vi "DAQmx_CreateAnalogPuls.vi"(0 "physical channel":string[](array[string])=["Dev1/ao0"], 5 "data":dbl[][](array[numeric]) format="%0.2f", 7 "rate":dbl=1000000.0, 11 "error in":errorcluster) -> (4 "task out":refnum<k21>, 15 "error out":errorcluster)   [LabVIEW 2010]
uses:
  <vilib>/DAQmx/write.llb/DAQmx Write.vi
  <vilib>/DAQmx/write.llb/DAQmx Write (Analog 2D DBL NChan NSamp).vi
  <vilib>/DAQmx/configure/timing.llb/DAQmx Timing (Sample Clock).vi
  <vilib>/DAQmx/configure/trigger.llb/DAQmx Trigger.vi
  <vilib>/DAQmx/configure/trigger.llb/DAQmx Start Trigger (Digital Edge).vi
  <vilib>/DAQmx/create/channels.llb/DAQmx Create Channel (AO-Voltage-Basic).vi
  <vilib>/daqmx/miscellaneous.llb/DAQmx Fill In Error Info.vi
  Program Files/National Instruments/LabVIEW 2010/resource/objmgr/daqmx.rc
panel:
  in  "timeout (s)":dbl=10.0 format="%0.2f"
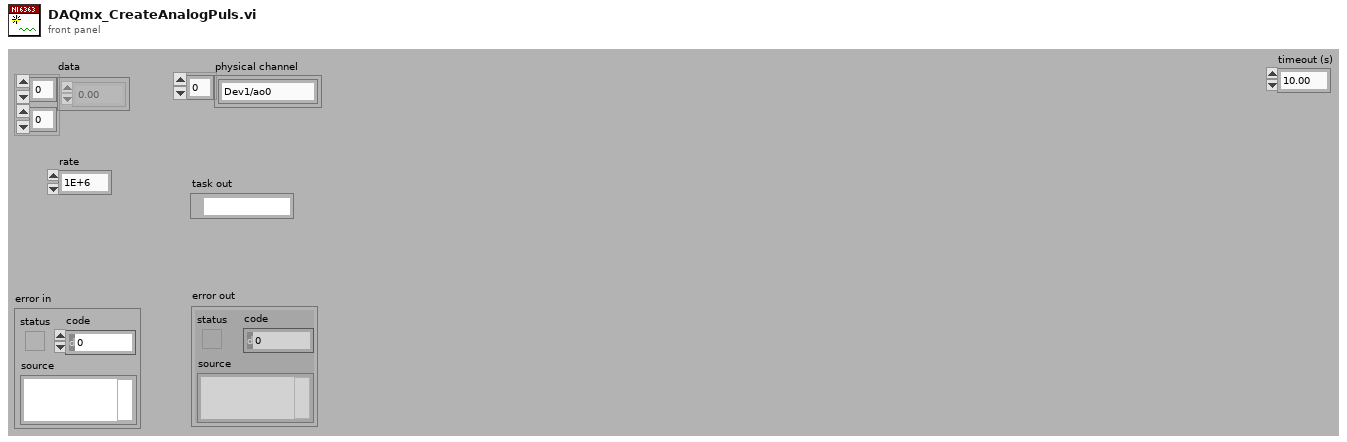
[diagram p1: front panel]
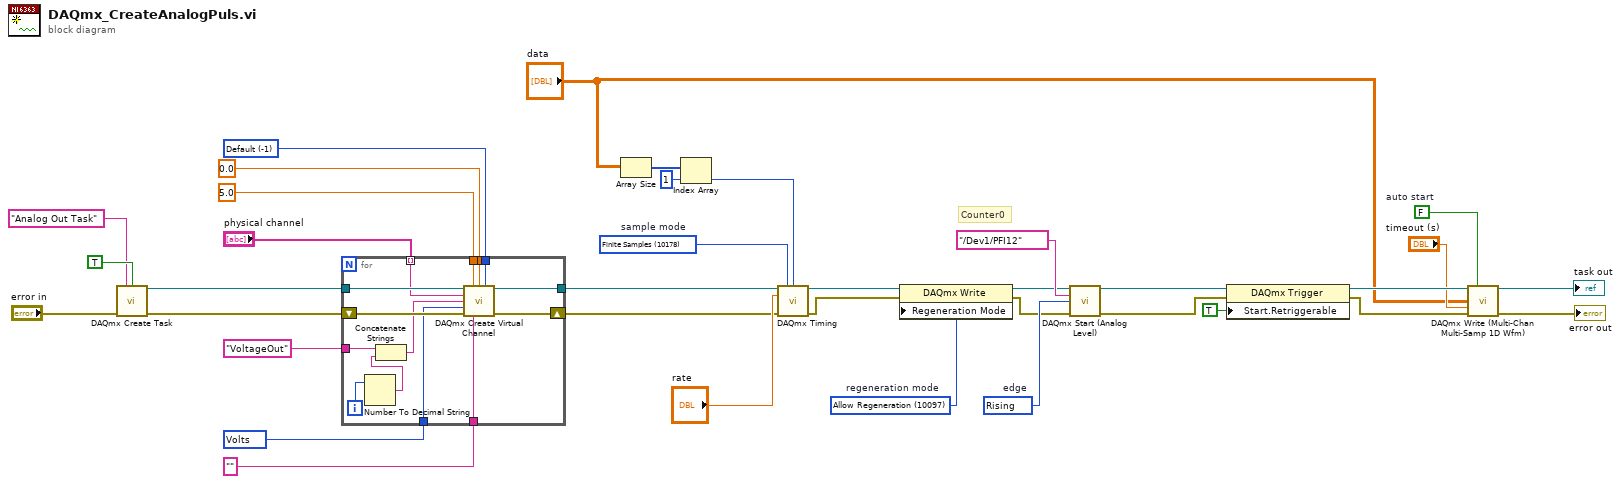
[diagram p0: block diagram]
diagram:
  w6 = -1 items=["Default"=-1, "RSE"=10083, "Differential"=10106, "Pseudodifferential"=12529] ("output terminal configuration")
  w10 = 10348 items=["Volts"=10348, "From Custom Scale"=10065] ("units")
  w15 = FALSE  # auto start
  w24 = 10280 items=["Rising"=10280, "Falling"=10171]  # edge
  w27 = 10097 items=["Allow Regeneration"=10097, "Do Not Allow Regeneration"=10158]  # regeneration mode
  w30 = 10178 items=["Finite Samples"=10178, "Continuous Samples"=10123, "Hardware Timed Single Point"=12522]  # sample mode
  # "Counter0"
  n1 = call <vilib>:"DAQmx Create Task.vi"("new task name"="Analog Out Task", "auto cleanup"=TRUE, "error in"="error in") -> ("task out"=w32:refnum<k21>, "error out"=w33:errorcluster)  [unwired: 11 in]
  n2 = for {
    tunnel: w32 -> [w50]
    tunnel: [w48] -> w28
    tunnel: 0.0 ("minimum value") -> [w46]
    tunnel: 5.0 ("maximum value") -> [w45]
    tunnel: "physical channel" -> [w44] mode=indexing
    tunnel: w10 -> [w43]
    tunnel: "" ("custom scale name") -> [w42]
    shift-right: [w47] -> w29
    shift-left: w33 -> [w49]
    tunnel: w6 -> [w41]
    tunnel: "VoltageOut" ("channel name") -> [w38]
    i -> [w39]
    n3 = Number To Decimal String(number=w39) -> (decimal integer string=w40:string)  [unwired: 1 in]
    n4 = Concatenate Strings(w38, w40) -> (w37:string)
    n5 = call-poly <vilib>:"DAQmx Create Virtual Channel.vi"("task in"=w50, "maximum value"=w45, "minimum value"=w46, "output terminal configuration"=w41, "physical channels"=w44, "name to assign"=w37, "units"=w43, "error in"=w49, "custom scale name"=w42) -> ("task out"=w48:refnum<k21>, "error out"=w47:errorcluster)  [unwired: 5 in]
  }
  n6 = Array Size(array="data") -> (size(s)=w5:i32[])
  n7 = Index Array(array=w5, index=1) -> (element=w3:i32)
  n8 = call-poly <vilib>:"DAQmx Timing.vi"("task/channels in"=w28, "sample mode"=w30, "samples per channel"=w3, "rate"="rate", "error in"=w29) -> ("task out"=w25:refnum<k21>, "error out"=w26:errorcluster)  [unwired: 9 in]
  n9 = property class="DAQmx Write"(reference=w25, error in=w26, "Regeneration Mode"=w27) -> (reference out=w19:refnum<k21>, error out=w18:errorcluster)
  n10 = call-poly "DAQmx Start (Analog Level).vi"("task/channels in"=w19, "source"=tag "/Dev1/PFI12", "edge"=w24, "error in"=w18) -> ("task out"=w23:refnum<k21>, "error out"=w22:errorcluster)  [unwired: 10 in]
  n11 = property class="DAQmx Trigger"(reference=w23, error in=w22, "Start.Retriggerable"=TRUE) -> (reference out=w17:refnum<k21>, error out=w16:errorcluster)
  n12 = call-poly "DAQmx Write (Multi-Chan Multi-Samp 1D Wfm).vi"("task/channels in"=w17, "auto start"=w15, "data"="data", "timeout"="timeout (s)", "error in"=w16) -> ("task out"=→"task out":refnum<k21>, "error out"=→"error out":errorcluster)  [unwired: 8 in, 1 out]
